vi "Повышенный уровень.vi"() -> ()   [LabVIEW 2024]
uses:
  <vilib>/addons/Modulation/niDMT.lvlib
panel:
  out "Хеш-код сообщения":i32
  out "?":picture
  out "LED-индикатордля проверки":bool
  out "Дешифрованный хеш-код":i32
  out "Хеш-код сообщения по модулю n":i32
  out "ЭЦП":i64
  out "СRC-16":i8[](array[numeric])
  out "?":picture
  out "Гамма":u64[](array[numeric])
  out "Вектор Sk":i32[](array[numeric])
  out "Вектор ключа K":i32[](array[numeric])
  out "Вектор S0":i32[](array[numeric])
  in  "Делитель 2":i32
  out "d":i32
  in  "e":i32
  in  "Делитель 1":i32
  out "new picture":picture
  in  "?":path
  # "Изображение после поточного шифрования"
  # "Дешифрованное изображение"
  # "Изначальное изображение"
  # "Поточное шифрование"
  # "Ввод параметров алгоритма RSA"
  # "Формирование ЭЦП"
  # "Большие простые делители числа n"
  # "Дешифрование ЭЦП"
  # "Полученное d"
  # "Если ЭЦП корректна, то индикатор загорится зеленым цветом"
  # "Вычисление хэш-кода CRC-16"
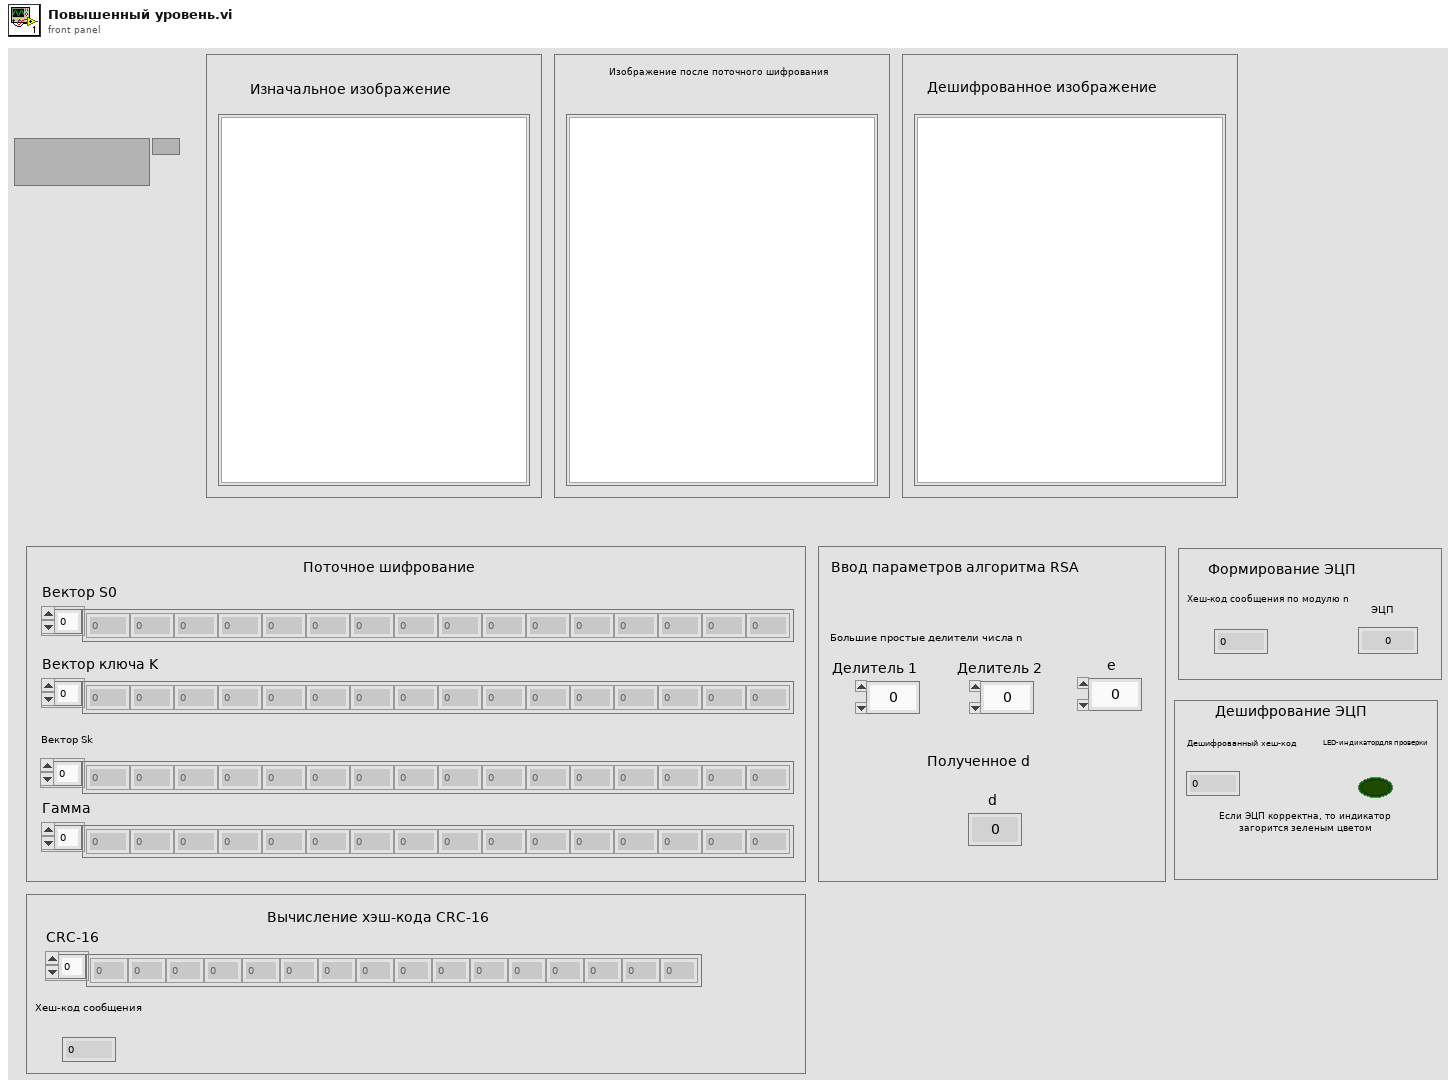
[diagram p1: front panel]
types:
  T1 = typedef "imagedata.ctl" = cluster{"image type":i32, "image depth":i32, "image":u8[], "mask":u8[], "colors":u32[], "Rectangle":cluster{"left":i16, "top":i16, "right":i16, "bottom":i16}}
  T2 = cluster{"left":i16, "top":i16, "right":i16, "bottom":i16}
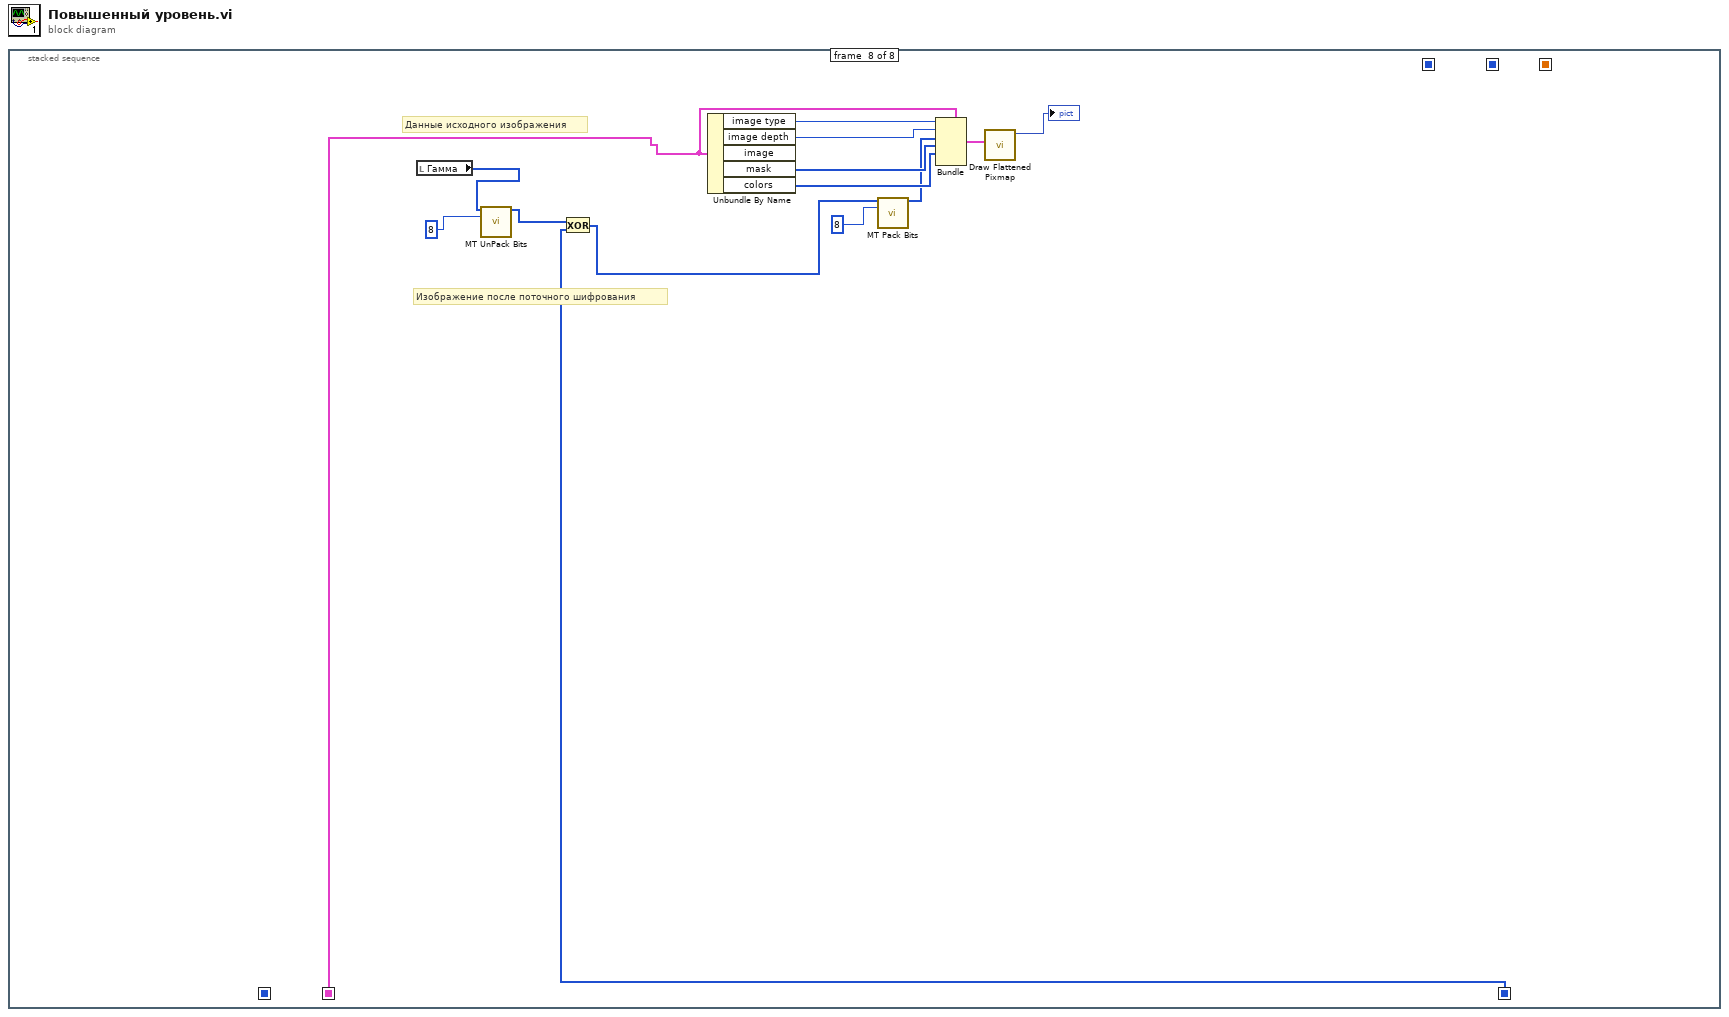
[diagram p0: block diagram]
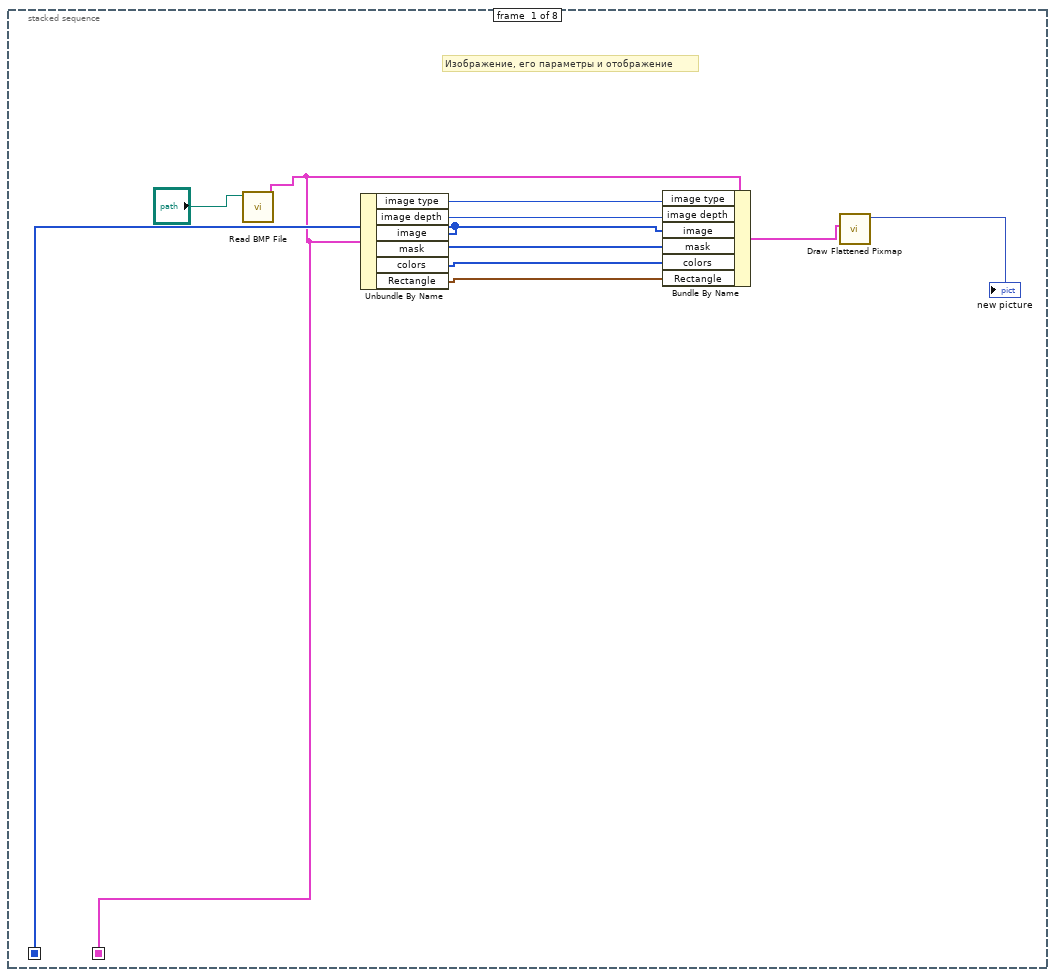
[diagram p2: hidden frame]
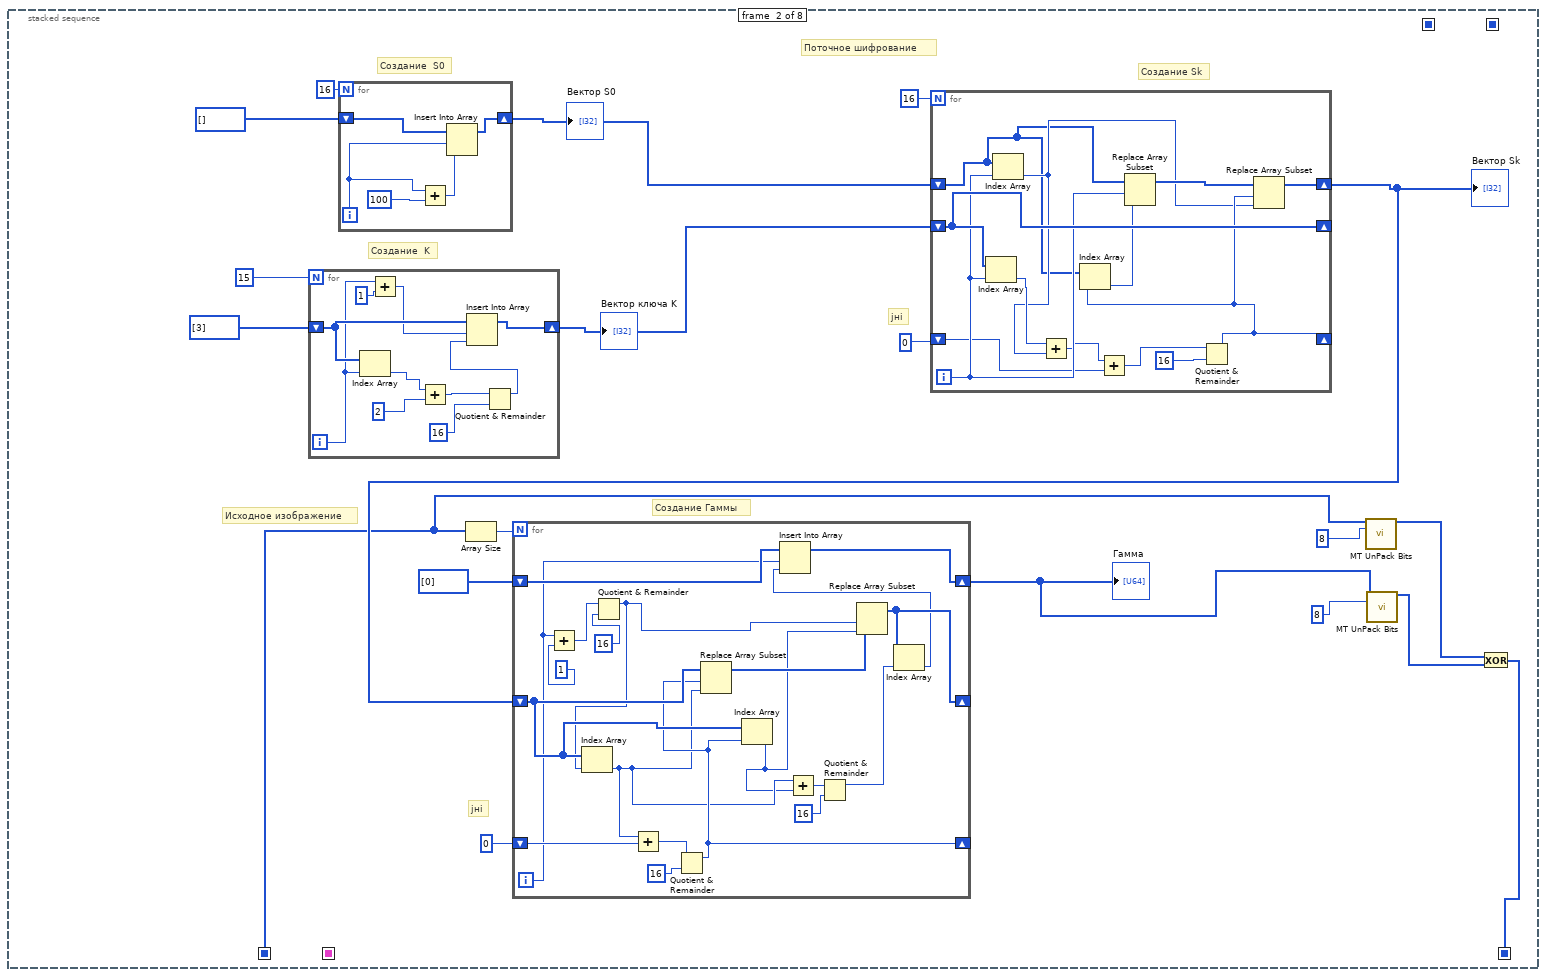
[diagram p3: hidden frame]
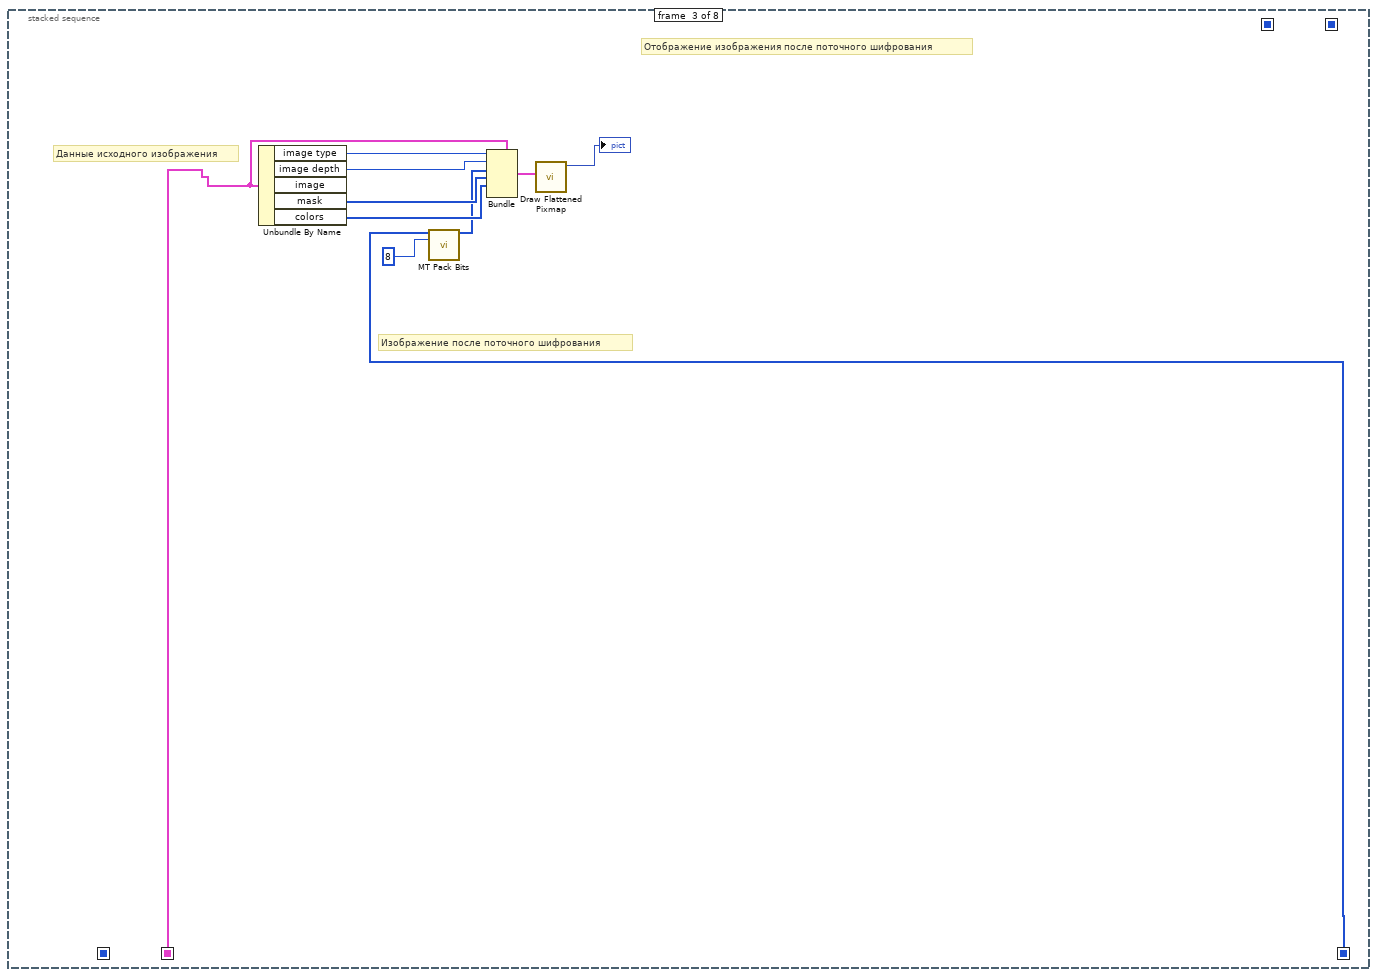
[diagram p4: hidden frame]
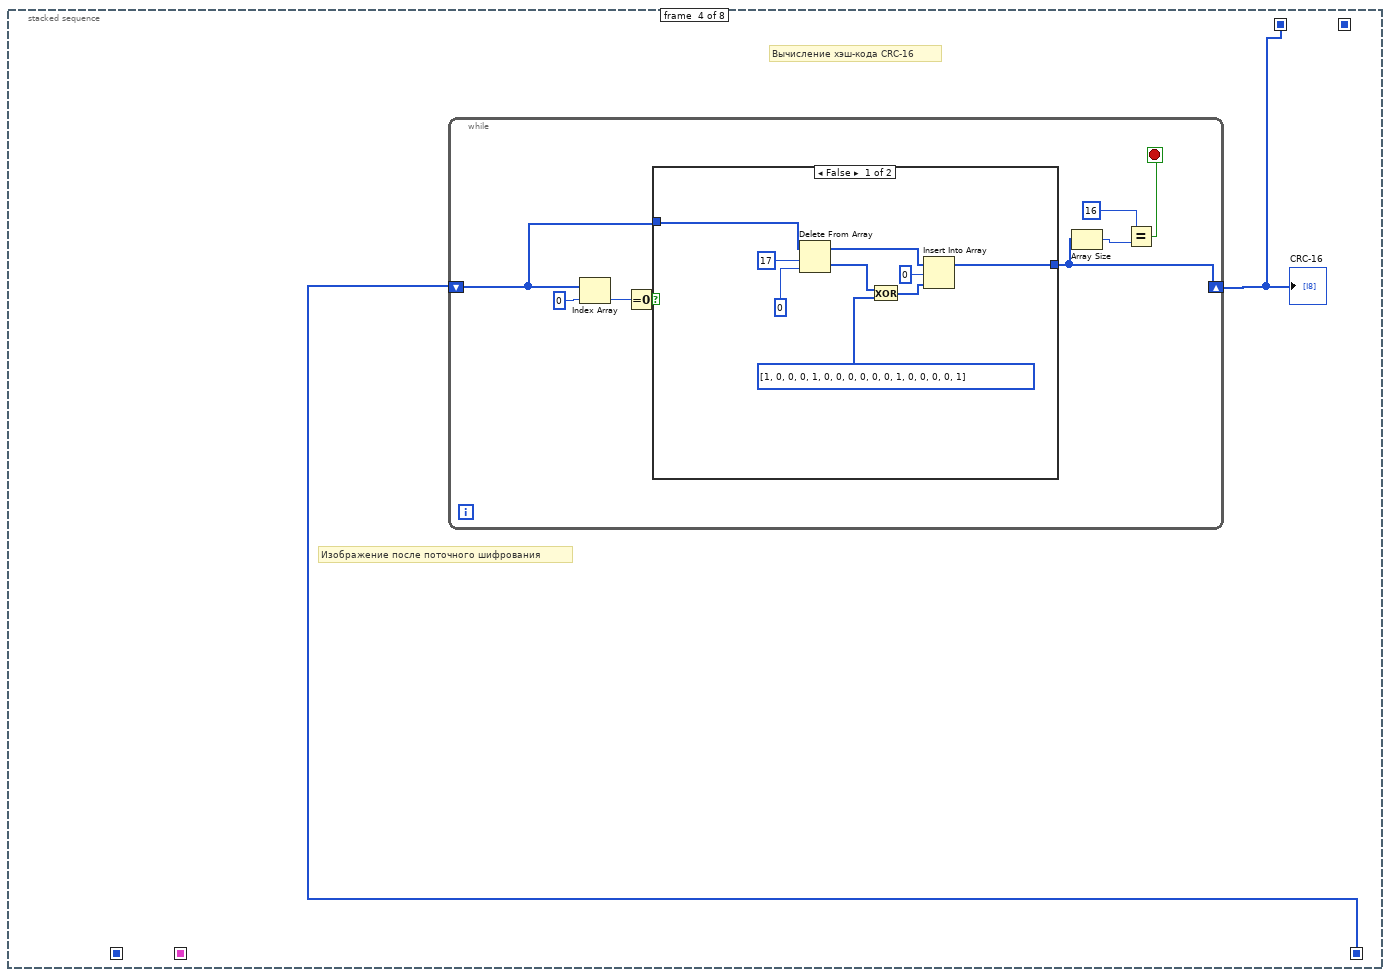
[diagram p5: hidden frame]
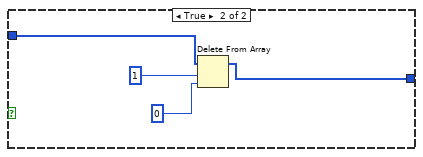
[diagram p6: hidden frame]
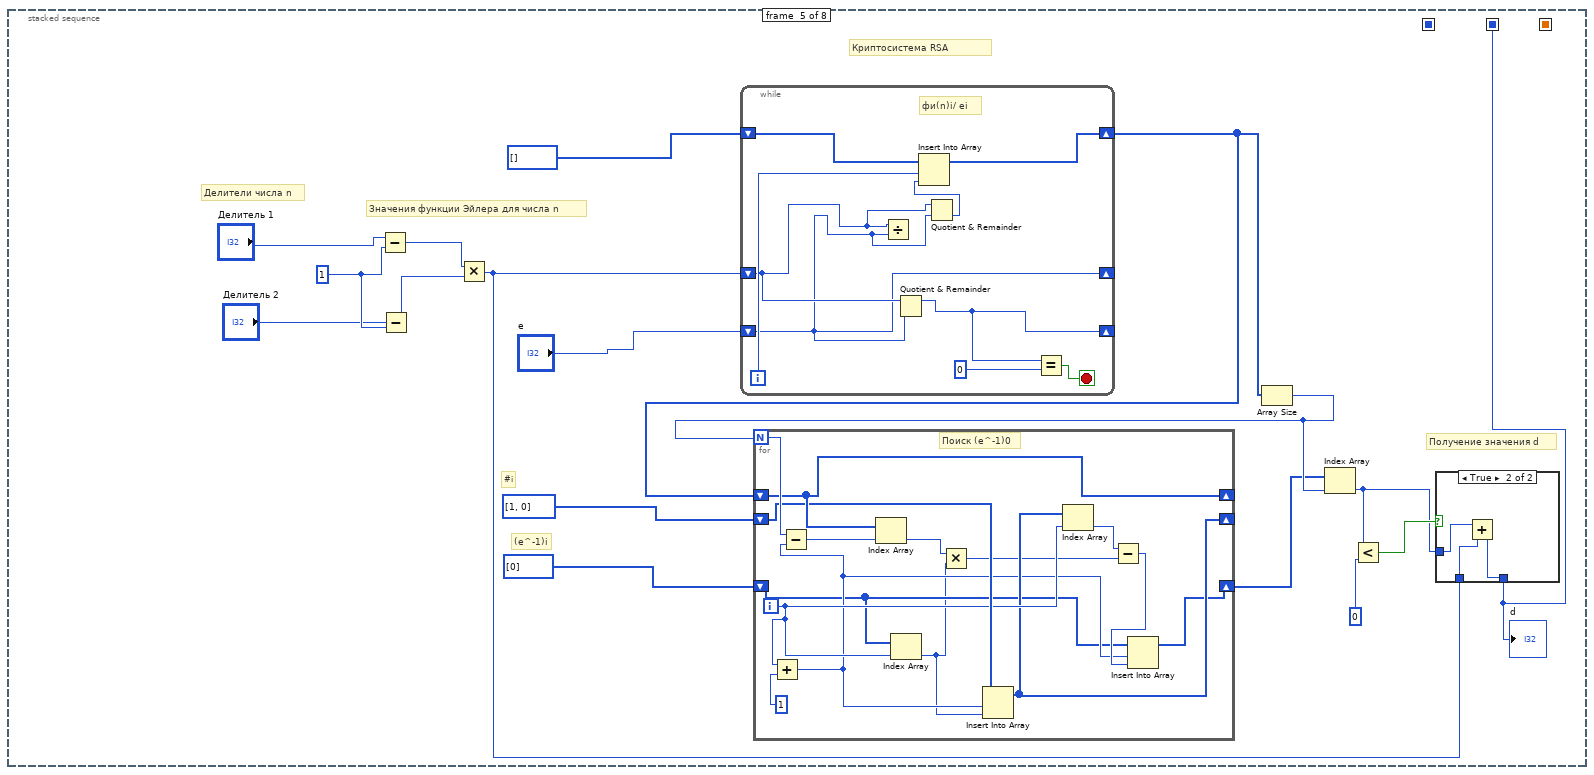
[diagram p7: hidden frame]
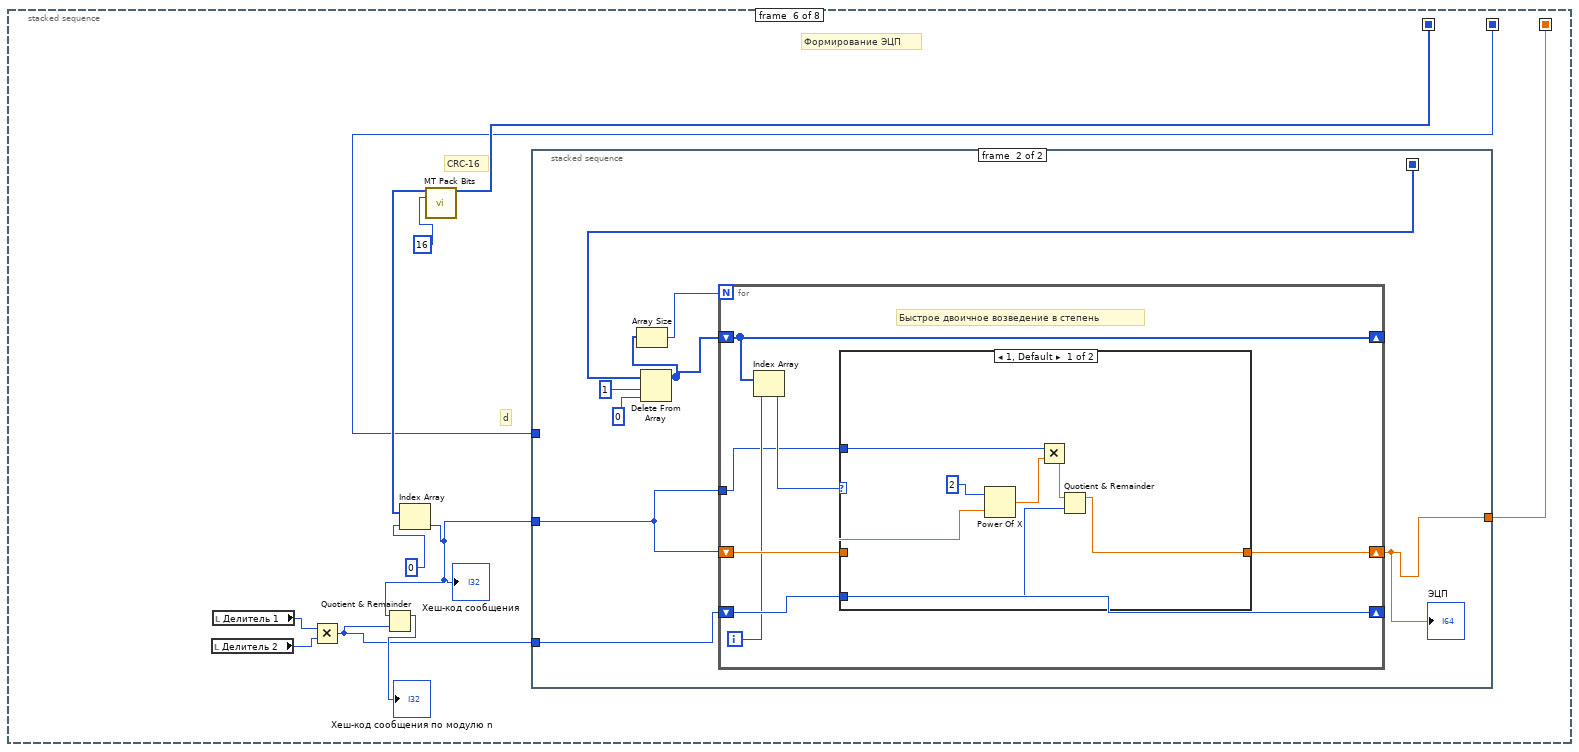
[diagram p9: hidden frame]
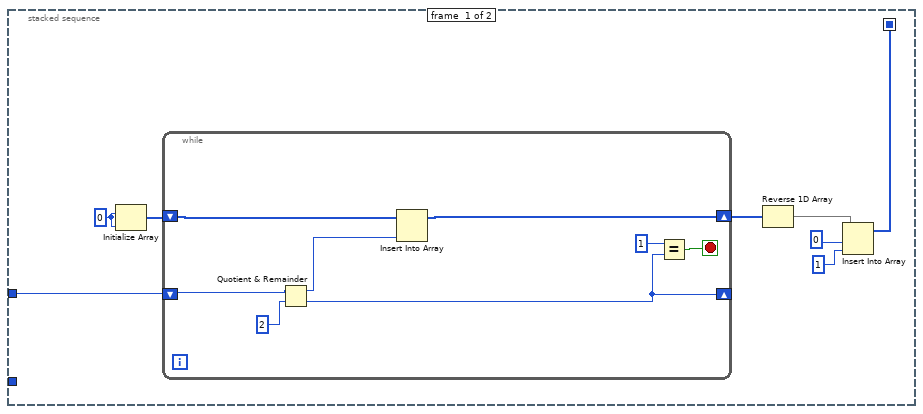
[diagram p10: hidden frame]
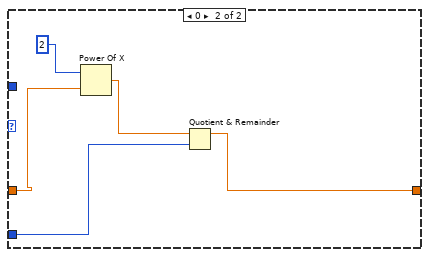
[diagram p11: hidden frame]
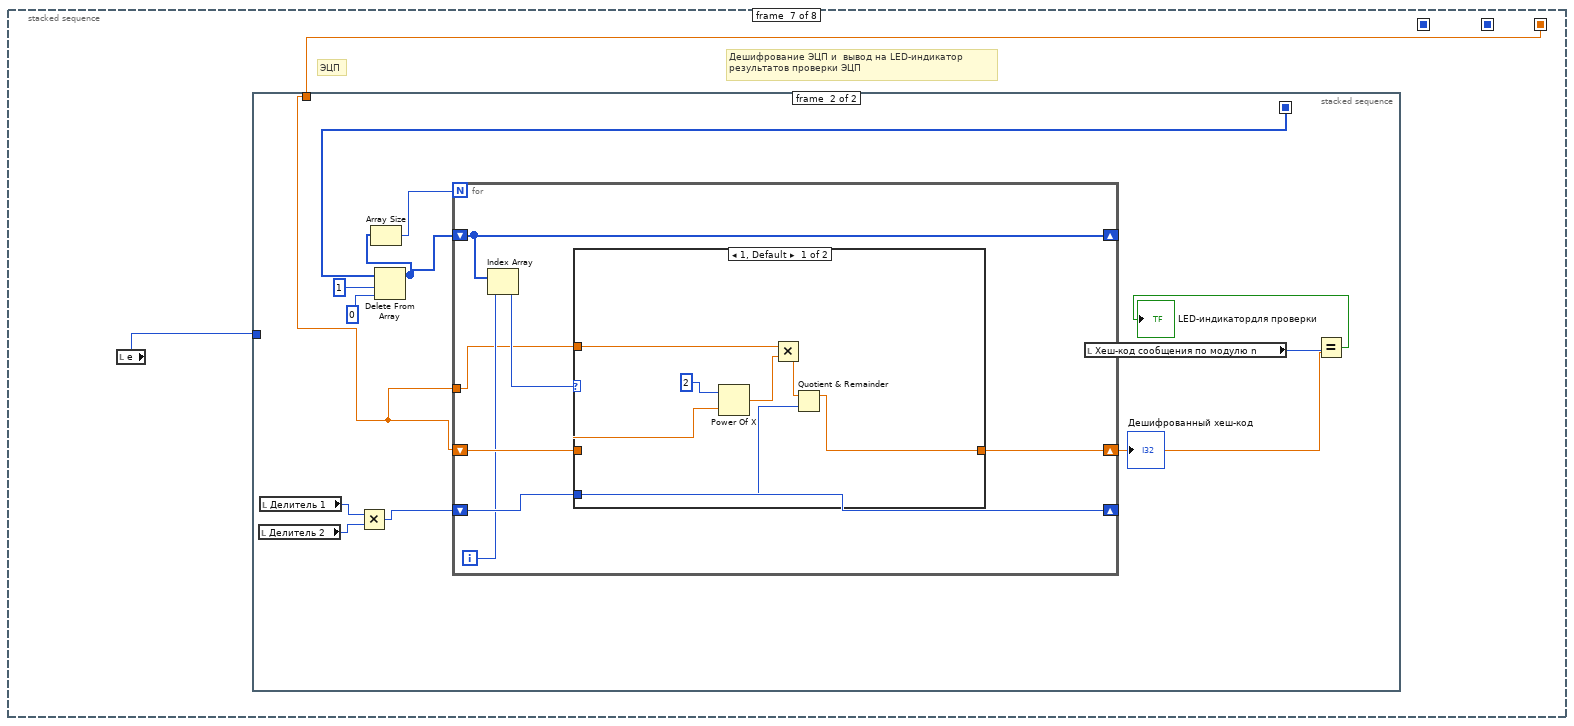
[diagram p12: hidden frame]
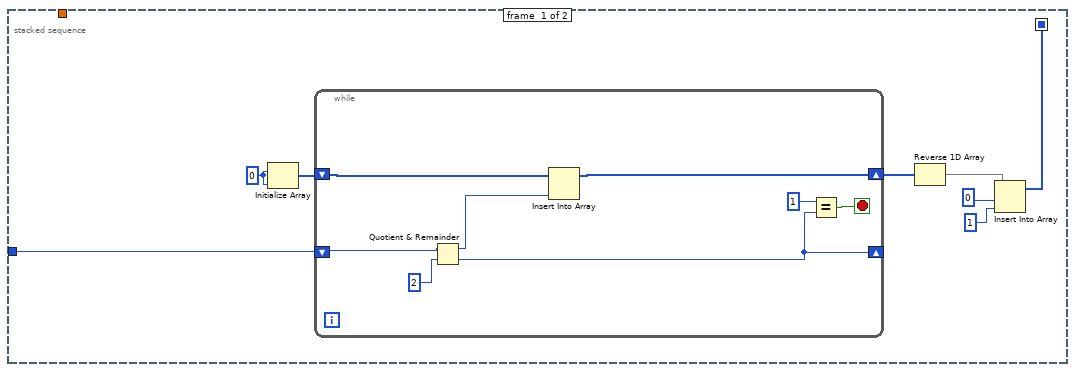
[diagram p13: hidden frame]
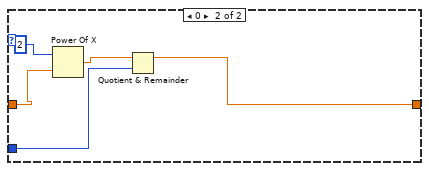
[diagram p14: hidden frame]
diagram:
  n1 = stacked-sequence {
    seq-local: [w2 _ _ _ _ _ _ _] -> [_ w14 _ _ _ _ _ _]
    seq-local: [w1 _ _ _ _ _ _ _] -> [_ _ w79 _ _ _ _ w262]
    seq-local: [_ w13 _ _ _ _ _ _] -> [_ _ w78 w89 _ _ _ w272]
    seq-local: [_ _ _ w88 _ _ _ _] -> [_ _ _ _ _ w163 _ _]
    seq-local: [_ _ _ _ w111 _ _ _] -> [_ _ _ _ _ w162 _ _]
    seq-local: [_ _ _ _ _ w160 _ _] -> [_ _ _ _ _ _ w210 _]
    frame #0 {
      # "Изображение, его параметры и отображение"
      n2 = call <vilib>:"Read BMP File.vi"("path to BMP file"="?") -> ("image data"=w1:T1)  [unwired: 8 in, 2 out]
      n3 = Unbundle By Name(w1) -> ("image type"=w9:i32, "image depth"=w8:i32, "image"=w2:u8[], "mask"=w7:u8[], "colors"=w6:u32[], "Rectangle"=w5:T2)
      n4 = Bundle By Name(cluster=w1, "image type"=w9, "image depth"=w8, "image"=w2, "mask"=w7, "colors"=w6, "Rectangle"=w5) -> (w4:T1)
      n5 = call <vilib>:"Draw Flattened Pixmap.vi"("image data"=w4) -> ("new picture"=→"new picture":picture)  [unwired: 8 in]
    }
    frame #1 {
      # "Исходное изображение"
      # "jнi"
      # "Поточное шифрование"
      # "Создание Гаммы"
      # "jнi"
      # "Создание Sk"
      # "Создание  K"
      # "Создание  S0"
      n6 = for {
        N: 15 -> [_]
        shift-right: [w66] -> w23
        shift-left: i32[] [3] -> [w67]
        i -> [w64]
        n7 = Index Array(array=w67, index=w64) -> (element=w71:i32)
        n8 = Add(x=w64, y=i64 1) -> (x+y=w63:i64)
        n9 = Add(x=w71, y=2) -> (x+y=w70:i32)
        n10 = Quotient & Remainder(x=w70, y=16) -> (x-y*floor(x/y)=w68:i32)  [unwired: 1 out]
        n11 = Insert Into Array(array=w67, index=w63, new element=w68) -> (w66:i32[])
      }
      "Вектор ключа K" <- w23
      n12 = for {
        N: 16 -> [_]
        shift-right: [w76] -> w24
        shift-left: i32[] [] -> [w77]
        i -> [w74]
        n13 = Add(x=w74, y=100) -> (x+y=w73:i32)
        n14 = Insert Into Array(array=w77, index=w74, new element=w73) -> (w76:i32[])
      }
      "Вектор S0" <- w24
      n15 = Array Size(array=w14) -> (size(s)=w20:i32)
      n16 = for {
        N: 16 -> [_]
        shift-right: [w57] -> w15
        shift-left: w24 -> [w50]
        shift-right: [w62] -> _
        shift-left: w23 -> [w62]
        shift-right: [w56] -> _
        shift-left: 0 -> [w52]
        i -> [w60]
        n17 = Index Array(array=w62, index=w60) -> (element=w55:i32)
        n18 = Index Array(array=w50, index=w60) -> (element=w54:i32)
        n19 = Add(x=w55, y=w54) -> (x+y=w53:i32)
        n20 = Add(x=w53, y=w52) -> (x+y=w51:i64)
        n21 = Quotient & Remainder(x=w51, y=i64 16) -> (x-y*floor(x/y)=w56:i64)  [unwired: 1 out]
        n22 = Index Array(array=w50, index=w56) -> (element=w59:i32)
        n23 = Replace Array Subset(array=w50, new element=w59, index=w60) -> (w58:i32[])
        n24 = Replace Array Subset(array=w58, new element=w54, index=w56) -> (w57:i32[])
      }
      "Вектор Sk" <- w15
      n25 = for {
        N: w20 -> [_]
        shift-right: [w35] -> _
        shift-left: w15 -> [w43]
        shift-right: [w41] -> _
        shift-left: 0 -> [w46]
        shift-right: [w30] -> w11
        shift-left: i32[] [0] -> [w33]
        i -> [w32]
        n26 = Add(x=w32, y=1) -> (x+y=w48:i32)
        n27 = Quotient & Remainder(x=w48, y=16) -> (x-y*floor(x/y)=w40:i32)  [unwired: 1 out]
        n28 = Index Array(array=w43, index=w40) -> (element=w37:i32)
        n29 = Add(x=w37, y=w46) -> (x+y=w45:i32)
        n30 = Quotient & Remainder(x=w45, y=16) -> (x-y*floor(x/y)=w41:i32)  [unwired: 1 out]
        n31 = Replace Array Subset(array=w43, new element=w37, index=w41) -> (w42:i32[])
        n32 = Index Array(array=w43, index=w41) -> (element=w36:i32)
        n33 = Add(x=w37, y=w36) -> (x+y=w39:i32)
        n34 = Quotient & Remainder(x=w39, y=16) -> (x-y*floor(x/y)=w34:i32)  [unwired: 1 out]
        n35 = Replace Array Subset(array=w42, new element=w36, index=w40) -> (w35:i32[])
        n36 = Index Array(array=w35, index=w34) -> (element=w31:i32)
        n37 = Insert Into Array(array=w33, index=w32, new element=w31) -> (w30:i32[])
      }
      "Гамма" <- w11
      n38 = call <vilib>:"MT UnPack Bits.vi"("input integers"=w14, "bits per integer"=8) -> ("output bit stream"=w19:i8[])  [unwired: 12 in, 1 out]
      n39 = call <vilib>:"MT UnPack Bits.vi"("input integers"=w11, "bits per integer"=8) -> ("output bit stream"=w18:i8[])  [unwired: 12 in, 1 out]
      n40 = Exclusive Or(1:w18, 2:w19) -> (0:w13:i8[])
    }
    frame #2 {
      # "Изображение после поточного шифрования"
      # "Данные исходного изображения"
      # "Отображение изображения после поточного шифрования"
      n41 = Unbundle By Name(w79) -> ("image type"=w87:i32, "image depth"=w84:i32, "mask"=w86:u8[], "colors"=w85:u32[])  [unwired: 1 out]
      n42 = call <vilib>:"MT Pack Bits.vi"("input bit stream"=w78, "bits per integer"=8) -> ("output integers"=w80:i32[])  [unwired: 12 in, 1 out]
      n43 = Bundle(cluster=w79, "image type"=w87, "image depth"=w84, "image"=w80, "mask"=w86, "colors"=w85) -> (w83:T1)  [unwired: 1 in]
      n44 = call <vilib>:"Draw Flattened Pixmap.vi"("image data"=w83) -> ("new picture"=→"?":picture)  [unwired: 8 in]
    }
    frame #3 {
      # "Изображение после поточного шифрования"
      # "Вычисление хэш-кода CRC-16"
      n45 = while {
        shift-right: [w93] -> w88
        shift-left: w89 -> [w94]
        stop <- w90 stop-if-true
        n46 = Index Array(array=w94, index=0) -> (element=w95:i8)
        n47 = Equal To 0?(x=w95) -> (x = 0?=w97:bool)
        n48 = case shown="False" w97 {
          tunnel: [w98 w107] -> w93
          tunnel: w94 -> [w106 w110]
          frame False {
            n49 = Delete From Array(array=w106, length=17, index=0 ("length")) -> (deleted portion=w102:i8[], array with subset deleted=w99:i8[])
            n50 = Exclusive Or(1:i32[] [1, 0, 0, 0, 1, 0, 0, 0, 0, 0, 0, 1, 0, 0, 0, 0, 1], 2:w102) -> (0:w101:i32[])
            n51 = Insert Into Array(array=w99, index=0, new element=w101) -> (w98:i8[])
          }
          frame True {
            n52 = Delete From Array(array=w110, length=1, index=0 ("length")) -> (array with subset deleted=w107:i8[])  [unwired: 1 out]
          }
        }
        n53 = Array Size(array=w93) -> (size(s)=w92:i32)
        n54 = Equal?(x=16, y=w92) -> (x = y?=w90:bool)
      }
      "СRC-16" <- w88
    }
    frame #4 {
      w127 = 1
      # "Получение значения d"
      # "(e^-1)i"
      # "#i"
      # "Значения функции Эйлера для числа n"
      # "Делители числа n"
      # "Криптосистема RSA"
      n55 = Subtract(x="Делитель 1", y=w127) -> (x-y=w125:i32)
      n56 = Subtract(x="Делитель 2", y=w127) -> (x-y=w126:i32)
      n57 = Multiply(x=w125, y=w126) -> (x*y=w112:i32)
      n58 = while {
        shift-right: [w148] -> _
        shift-left: w112 -> [w149]
        shift-right: [w150] -> _
        shift-left: "e" -> [w148]
        shift-right: [w151] -> w123
        shift-left: i32[] [] -> [w152]
        i -> [w153]
        stop <- w155 stop-if-true
        # "фи(n)i/ еi"
        n59 = Divide(x=w149, y=w148) -> ()  [unwired: 1 out]
        n60 = Quotient & Remainder(x=w149, y=w148) -> (x-y*floor(x/y)=w150:i32)  [unwired: 1 out]
        n61 = Quotient & Remainder(x=w149, y=w148) -> (floor(x/y)=w147:i32)  [unwired: 1 out]
        n62 = Insert Into Array(array=w152, index=w153, new element=w147) -> (w151:i32[])
        n63 = Equal?(x=w150, y=0) -> (x = y?=w155:bool)
      }
      n64 = Array Size(array=w123) -> (size(s)=w120:i32)
      n65 = for {
        N: w120 -> [w146]
        shift-right: [w139] -> _
        shift-left: i32[] [1, 0] -> [w142]
        shift-right: [w133] -> w119
        shift-left: i32[] [0] -> [w134]
        shift-right: [w145] -> _
        shift-left: w123 -> [w145]
        i -> [w140]
        # "Поиск (e^-1)0"
        n66 = Add(x=w140, y=i64 1) -> (x+y=w135:i64)
        n67 = Subtract(x=w146, y=w135) -> (x-y=w143:i64)
        n68 = Index Array(array=w145, index=w143) -> (element=w141:i32)
        n69 = Index Array(array=w134, index=w140) -> (element=w132:i32)
        n70 = Multiply(x=w141, y=w132) -> (x*y=w137:i32)
        n71 = Insert Into Array(array=w142, index=w135, new element=w132) -> (w139:i32[])
        n72 = Index Array(array=w139, index=w140) -> (element=w138:i32)
        n73 = Subtract(x=w138, y=w137) -> (x-y=w136:i32)
        n74 = Insert Into Array(array=w134, index=w135, new element=w136) -> (w133:i32[])
      }
      n75 = Index Array(array=w119, index=w120) -> (element=w113:i32)
      n76 = Less?(x=w113, y=i64 0) -> (x < y?=w114:bool)
      n77 = case shown="True" w114 {
        tunnel: w113 -> [w128 w130]
        tunnel: w112 -> [_ w131]
        tunnel: [w128 w129] -> w111
        frame False {
        }
        frame True {
          n78 = Add(x=w130, y=w131) -> (x+y=w129:i32)
        }
      }
      "d" <- w111
    }
    frame #5 {
      # "d"
      # "CRC-16"
      # "Формирование ЭЦП"
      n79 = local read "Делитель 2"() -> (w159:i32)
      n80 = local read "Делитель 1"() -> (w158:i32)
      n81 = Multiply(x=w158, y=w159) -> (x*y=w157:i32)
      n82 = call <vilib>:"MT Pack Bits.vi"("input bit stream"=w163, "bits per integer"=16) -> ("output integers"=w166:i32[])  [unwired: 12 in, 1 out]
      n83 = Index Array(array=w166, index=0) -> (element=w156:i32)
      "Хеш-код сообщения" <- w156
      n84 = Quotient & Remainder(x=w156, y=w157) -> (x-y*floor(x/y)=→"Хеш-код сообщения по модулю n":i32)  [unwired: 1 out]
      n85 = stacked-sequence {
        seq-local: [w168 _] -> [_ w188]
        tunnel: w162 -> [w167 _]
        tunnel: w156 -> [_ w185]
        tunnel: [_ w184] -> w160
        tunnel: w157 -> [_ w183]
        frame #0 {
          w174 = 0 ("dimension size")
          n86 = Initialize Array(w174, w174) -> (w173:i32[])
          n87 = while {
            shift-right: [w175] -> _
            shift-left: w167 -> [w180]
            shift-right: [w176] -> w171
            shift-left: w173 -> [w178]
            stop <- w181 stop-if-true
            n88 = Quotient & Remainder(x=w180, y=2) -> (x-y*floor(x/y)=w177:i32, floor(x/y)=w175:i32)
            n89 = Insert Into Array(array=w178, new element=w177) -> (w176:i32[])  [unwired: 1 in]
            n90 = Equal?(x=1, y=w175) -> (x = y?=w181:bool)
          }
          n91 = Reverse 1D Array(array=w171) -> (reversed array=w170:i32[])
          n92 = Insert Into Array(array=w170, index=0 ("new element/subarray"), new element=1 ("new element/subarray")) -> (w168:i32[])
        }
        frame #1 {
          n93 = Delete From Array(array=w188, length=1 ("index"), index=0) -> (array with subset deleted=w186:i32[])  [unwired: 1 out]
          n94 = Array Size(array=w186) -> (size(s)=w187:i32)
          n95 = for {
            N: w187 -> [_]
            shift-right: [w195] -> w184
            shift-left: w185 -> [w197]
            shift-right: [w196] -> _
            shift-left: w183 -> [w196]
            shift-right: [w192] -> _
            shift-left: w186 -> [w192]
            tunnel: w185 -> [w191]
            i -> [w194]
            # "Быстрое двоичное возведение в степень"
            n96 = Index Array(array=w192, index=w194) -> (element=w193:i32)
            n97 = case shown="1, Default" w193 {
              tunnel: w197 -> [w203 w209]
              tunnel: w196 -> [w202 w208]
              tunnel: [w201 w206] -> w195
              tunnel: w191 -> [w200 _]
              frame 1, Default {
                n98 = Power Of X(1:w203, 2:2) -> (0:w199:dbl)
                n99 = Multiply(x=w200, y=w199) -> (x*y=w198:dbl)
                n100 = Quotient & Remainder(x=w198, y=w202) -> (x-y*floor(x/y)=w201:dbl)  [unwired: 1 out]
              }
              frame 0 {
                n101 = Power Of X(1:w209, 2:2) -> (0:w207:dbl)
                n102 = Quotient & Remainder(x=w207, y=w208) -> (x-y*floor(x/y)=w206:dbl)  [unwired: 1 out]
              }
            }
          }
          "ЭЦП" <- w184
        }
      }
    }
    frame #6 {
      # "ЭЦП"
      # "Дешифрование ЭЦП и  вывод на LED-индикатор\nрезультатов проверки ЭЦП"
      n103 = local read "e"() -> (w211:i32)
      n104 = stacked-sequence {
        seq-local: [w213 _] -> [_ w237]
        tunnel: w211 -> [w212 _]
        tunnel: w210 -> [_ w234]
        frame #0 {
          w219 = 0 ("dimension size")
          n105 = Initialize Array(w219, w219) -> (w218:i32[])
          n106 = while {
            shift-right: [w220] -> _
            shift-left: w212 -> [w225]
            shift-right: [w221] -> w216
            shift-left: w218 -> [w223]
            stop <- w226 stop-if-true
            n107 = Quotient & Remainder(x=w225, y=2) -> (x-y*floor(x/y)=w222:i32, floor(x/y)=w220:i32)
            n108 = Insert Into Array(array=w223, new element=w222) -> (w221:i32[])  [unwired: 1 in]
            n109 = Equal?(x=1, y=w220) -> (x = y?=w226:bool)
          }
          n110 = Reverse 1D Array(array=w216) -> (reversed array=w215:i32[])
          n111 = Insert Into Array(array=w215, index=0 ("new element/subarray"), new element=1 ("new element/subarray")) -> (w213:i32[])
        }
        frame #1 {
          n112 = local read "Делитель 2"() -> (w232:i32)
          n113 = local read "Делитель 1"() -> (w233:i32)
          n114 = Multiply(x=w233, y=w232) -> (x*y=w231:i32)
          n115 = Delete From Array(array=w237, length=1 ("index"), index=0) -> (array with subset deleted=w235:i32[])  [unwired: 1 out]
          n116 = Array Size(array=w235) -> (size(s)=w236:i32)
          n117 = for {
            N: w236 -> [_]
            shift-right: [w244] -> w228
            shift-left: w234 -> [w246]
            shift-right: [w245] -> _
            shift-left: w231 -> [w245]
            shift-right: [w241] -> _
            shift-left: w235 -> [w241]
            tunnel: w234 -> [w240]
            i -> [w243]
            n118 = Index Array(array=w241, index=w243) -> (element=w242:i32)
            n119 = case shown="1, Default" w242 {
              tunnel: w246 -> [w252 w258]
              tunnel: w245 -> [w251 w257]
              tunnel: [w250 w255] -> w244
              tunnel: w240 -> [w249 _]
              frame 1, Default {
                n120 = Power Of X(1:w252, 2:2) -> (0:w248:dbl)
                n121 = Multiply(x=w249, y=w248) -> (x*y=w247:dbl)
                n122 = Quotient & Remainder(x=w247, y=w251) -> (x-y*floor(x/y)=w250:dbl)  [unwired: 1 out]
              }
              frame 0 {
                n123 = Power Of X(1:w258, 2:2) -> (0:w256:dbl)
                n124 = Quotient & Remainder(x=w256, y=w257) -> (x-y*floor(x/y)=w255:dbl)  [unwired: 1 out]
              }
            }
          }
          "Дешифрованный хеш-код" <- w228
          n125 = local read "Хеш-код сообщения по модулю n"() -> (w229:i32)
          n126 = Equal?(x=w229, y=w228) -> (x = y?=→"LED-индикатордля проверки":bool)
        }
      }
    }
    frame #7 {
      # "Данные исходного изображения"
      # "Изображение после поточного шифрования"
      n127 = local read "Гамма"() -> (w260:u64[])
      n128 = call <vilib>:"MT UnPack Bits.vi"("input integers"=w260, "bits per integer"=8) -> ("output bit stream"=w259:i8[])  [unwired: 12 in, 1 out]
      n129 = Exclusive Or(1:w272, 2:w259) -> (0:w263:i8[])
      n130 = Unbundle By Name(w262) -> ("image type"=w271:i32, "image depth"=w268:i32, "mask"=w270:u8[], "colors"=w269:u32[])  [unwired: 1 out]
      n131 = call <vilib>:"MT Pack Bits.vi"("input bit stream"=w263, "bits per integer"=8) -> ("output integers"=w264:i32[])  [unwired: 12 in, 1 out]
      n132 = Bundle(cluster=w262, "image type"=w271, "image depth"=w268, "image"=w264, "mask"=w270, "colors"=w269) -> (w267:T1)  [unwired: 1 in]
      n133 = call <vilib>:"Draw Flattened Pixmap.vi"("image data"=w267) -> ("new picture"=→"?":picture)  [unwired: 8 in]
    }
  }
